vi "Login.vi"(7 "error in":errorcluster caption="error in (no error)") -> (0 "error out":errorcluster, 2 "OK?":bool caption="OK", 3 "Level":T1(ring))   [LabVIEW 2019, in "GUI.lvlib"]
doc: "Displays a standard dialog box that prompts users to enter information, such as a user name and password.\n--------------------\n\nThis Express VI is configured as follows:\n\nMessage to Display to the User:\nThe inputs are:"
uses:
  GUI.lvlib
  Controls/User Info.ctl
panel:
  in  "User":string(combo)="Engineer" caption="Default Pattern Folder"
  in  "Password":string
  in  "Cancel":bool
  in  "OK":bool caption="OK2"
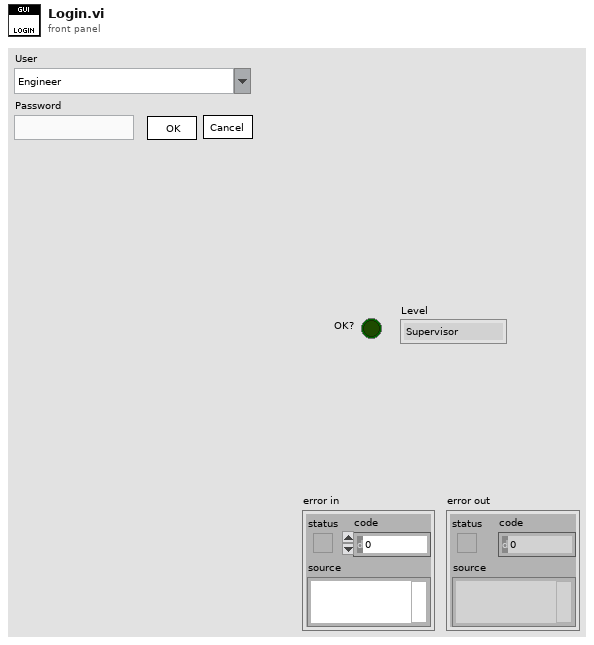
[diagram p1: front panel]
types:
  T1 = enum16{"Supervisor", "Engineer", "Operator", "Guest"}
  T2 = typedef "GUI.lvlib/User Info.ctl" = cluster{"ID":string, "Password":string, "Level":enum16{"Supervisor", "Engineer", "Operator", "Guest"}}[]
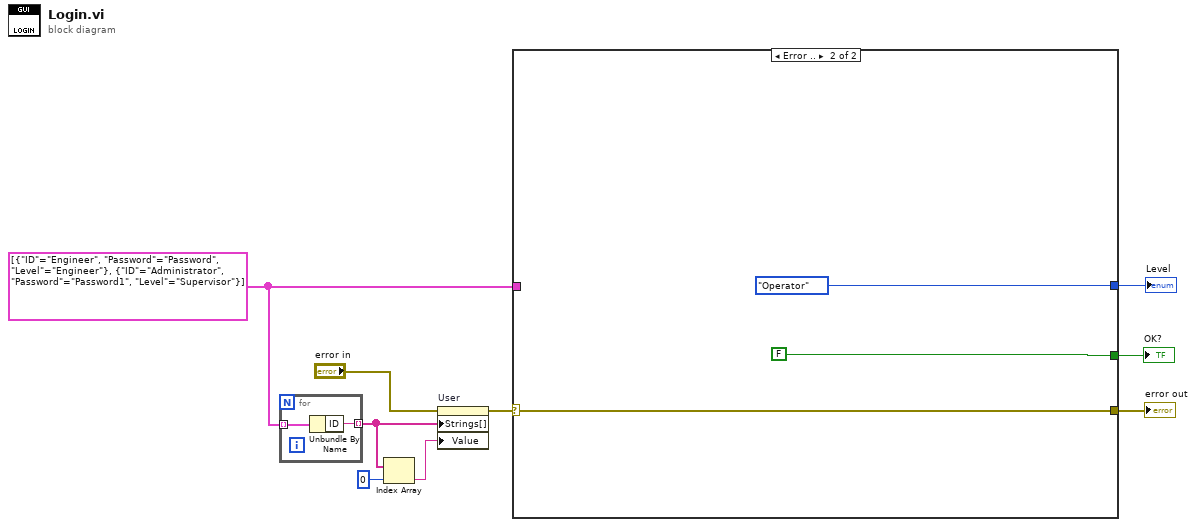
[diagram p0: block diagram]
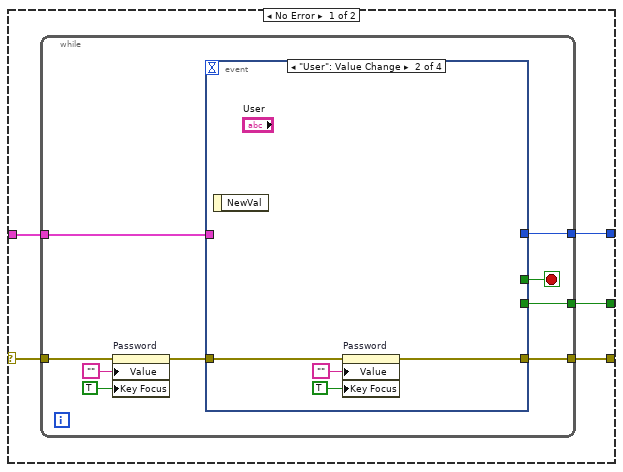
[diagram p2: hidden frame]
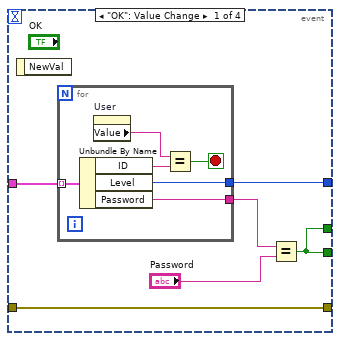
[diagram p3: hidden frame]
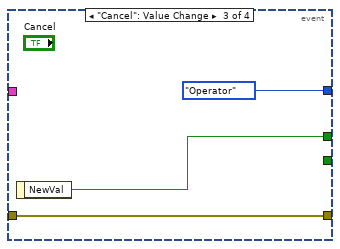
[diagram p4: hidden frame]
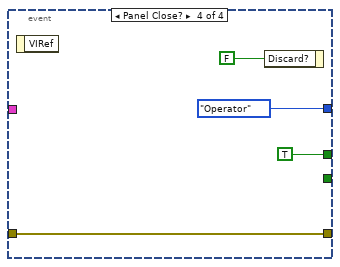
[diagram p5: hidden frame]
diagram:
  w1 = T2 [{"ID"="Engineer", "Password"="Password", "Level"=enum."Engineer"}, {"ID"="Administrator", "Password"="Password1", "Level"=enum."Supervisor"}] ("User List")
  n1 = for {
    tunnel: w1 -> [w11] mode=indexing
    tunnel: [w10] -> w5 mode=indexing
    n2 = Unbundle By Name(w11) -> ("ID"=w10:string)
  }
  n3 = Index Array(array=w5, index=0) -> (element=w4:string)
  n4 = property on="User" class="CmbBox"(error in="error in", "Strings[]"=w5, "Value"=w4) -> (error out=w3:errorcluster)  [unwired: 1 in, 1 out]
  n5 = case shown="Error .." w3 {
    selector: w3 -> [w15 w51]
    tunnel: [w13 FALSE] -> w9
    tunnel: [w16 w51] -> w8
    tunnel: w1 -> [w14 _]
    tunnel: [w12 T1."Operator" ("Level")] -> w7
    frame No Error {
      n6 = while "Main While Loop" {
        tunnel: w15 -> [w18]
        tunnel: [w21] -> w16
        tunnel: w14 -> [w24]
        tunnel: [w23] -> w13
        tunnel: [w22] -> w12
        stop <- w25 stop-if-true
        n7 = property on="Password" class="Str"(error in=w18, "Value"="", "Key Focus"=TRUE) -> (error out=w17:errorcluster)  [unwired: 1 in, 1 out]
        n8 = event shown="[1] \"User\": Value Change" {
          selector: _ -> [_ _ _ _]
          dyn-events: _ -> [_ _ _ _]
          timeout: _ -> [_ _ _ _]
          tunnel: [w28 _ w44 TRUE ("NewVal")] -> w25
          tunnel: w17 -> [w31 w39 w43 w46]
          tunnel: [w31 w38 w43 w46] -> w21
          tunnel: w24 -> [w30 _ _ _]
          tunnel: [w28 _ _ _] -> w23
          tunnel: [w27 _ T1."Operator" ("f") T1."Operator" ("f")] -> w22
          event "OK": Value Change {
            n9 = event-data() -> ()  [unwired: 1 in, 1 out]
            n10 = for {
              tunnel: w30 -> [w37] mode=indexing
              tunnel: [w33] -> w29
              tunnel: [w32] -> w27
              stop <- w34 stop-if-true
              n11 = Unbundle By Name(w37) -> ("ID"=w36:string, "Level"=w32:T1, "Password"=w33:string)
              n12 = property on="User" class="CmbBox"() -> ("Value"=w35:string)  [unwired: 2 in, 2 out]
              n13 = Equal?(x=w35, y=w36) -> (x = y?=w34:bool)
            }
            n14 = Equal?(x=w29, y="Password") -> (x = y?=w28:bool)
          }
          event "User": Value Change {
            n15 = event-data() -> ()  [unwired: 1 in, 1 out]
            n16 = property on="Password" class="Str"(error in=w39, "Value"="", "Key Focus"=TRUE) -> (error out=w38:errorcluster)  [unwired: 1 in, 1 out]
          }
          event "Cancel": Value Change {
            n17 = event-data() -> ("NewVal"=w44:bool)  [unwired: 1 in]
          }
          event Panel Close? {
            n18 = event-data() -> ()  [unwired: 1 in, 1 out]
            n19 = event-data("Discard?"=FALSE) -> ()  [unwired: 1 in, 1 out]
          }
        }
      }
    }
    frame Error {
    }
  }
  "OK?" <- w9
  "error out" <- w8
  "Level" <- w7
